vi "MatchInputTypes.vi"() -> ()   [LabVIEW 2013]
uses:
  <vilib>/Utility/VariantDataType/VariantType.lvlib
panel:
  out "Inputs":variant
  out "Input type":variant
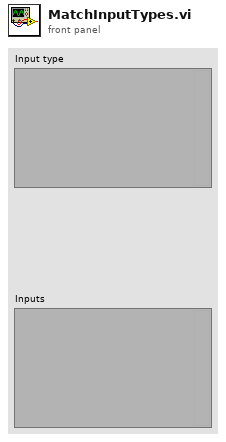
[diagram p1: front panel]
types:
  T1 = typedef "VariantType.lvlib/Type.ctl" = enum8{"Invalid Type", "Void", "I8", "I16", "I32", "I64", "U8", "U16", "U32", "U64", "Single Float", "Double Float", "Extended Float", "Single Complex", "Double Complex", "Extended Complex", "Enum U8", "Enum U16", "Enum U32", "Enum U64", "Single Float With Unit", "Double Float With Unit", "Extended Float With Unit", "Single Complex with Unit", "Double Complex with Unit", "Extended Complex with Unit", "Boolean", "String", "Path", "Picture", "Tag", "Array", "Cluster", "Variant", "LV Variant", "Waveform", "Timestamp", "Digital Waveform", "Digital Data", "ExpressData", "Refnum", "External Data", "VI", "Poly VI", "LabVIEW Class Instance", "Fixed Point"}
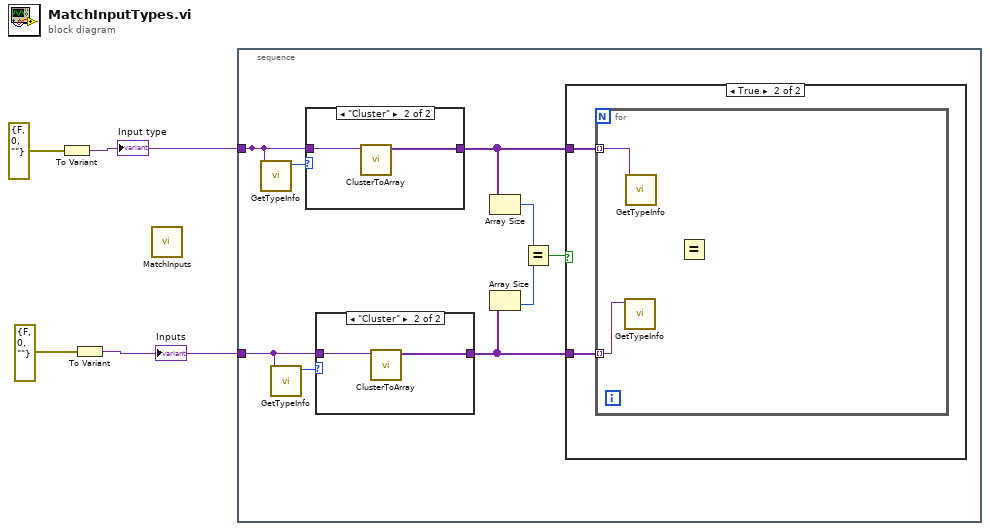
[diagram p0: block diagram]
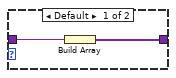
[diagram p3: hidden frame]
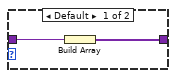
[diagram p4: hidden frame]
diagram:
  n1 = To Variant(anything=errorcluster {"status"=FALSE, "code"=0, "source"=""} ("error constant")) -> (Variant=w2:variant)
  "Input type" <- w2
  n2 = To Variant(anything=errorcluster {"status"=FALSE, "code"=0, "source"=""} ("error constant")) -> (Variant=w1:variant)
  "Inputs" <- w1
  n3 = call "MatchInputs.vi"() -> ()  [unwired: 10 in, 2 out]
  n4 = stacked-sequence {
    tunnel: w2 -> [w5]
    tunnel: w1 -> [w6]
    frame #0 {
      n5 = call <vilib>:"GetTypeInfo.vi"("Variant"=w5) -> ("Type Enum"=w13:T1)  [unwired: 6 in, 4 out]
      n6 = call <vilib>:"GetTypeInfo.vi"("Variant"=w6) -> ("Type Enum"=w12:T1)  [unwired: 6 in, 4 out]
      n7 = case shown="\"Cluster\"" w13 {
        tunnel: w5 -> [w23 w25]
        tunnel: [w22 w24] -> w9
        frame Default {
          n8 = Build Array(w23) -> (w22:variant[])
        }
        frame "Cluster" {
          n9 = call "ClusterToArray.vi"("Cluster"=w25) -> ("Array"=w24:variant[])  [unwired: 10 in]
        }
      }
      n10 = case shown="\"Cluster\"" w12 {
        tunnel: w6 -> [w19 w21]
        tunnel: [w18 w20] -> w8
        frame Default {
          n11 = Build Array(w19) -> (w18:variant[])
        }
        frame "Cluster" {
          n12 = call "ClusterToArray.vi"("Cluster"=w21) -> ("Array"=w20:variant[])  [unwired: 10 in]
        }
      }
      n13 = Array Size(array=w9) -> (size(s)=w11:i32)
      n14 = Array Size(array=w8) -> (size(s)=w10:i32)
      n15 = Equal?(x=w11, y=w10) -> (x = y?=w7:bool)
      n16 = case shown="True" w7 {
        tunnel: w9 -> [_ w15]
        tunnel: w8 -> [_ w14]
        frame False {
        }
        frame True {
          n17 = for {
            tunnel: w15 -> [w17] mode=indexing
            tunnel: w14 -> [w16] mode=indexing
            n18 = call <vilib>:"GetTypeInfo.vi"("Variant"=w16) -> ()  [unwired: 6 in, 5 out]
            n19 = call <vilib>:"GetTypeInfo.vi"("Variant"=w17) -> ()  [unwired: 6 in, 5 out]
            n20 = Equal?() -> ()  [unwired: 2 in, 1 out]
          }
        }
      }
    }
  }
